vi "Restore X & Scale Indices.vi"(5 "New Plot Style in":T1, 9 "Original Plot Style in":T1) -> (8 "Updated Plot Style out":T1)   [LabVIEW 2019]
uses:
  XY Graph Plot Properties.ctl
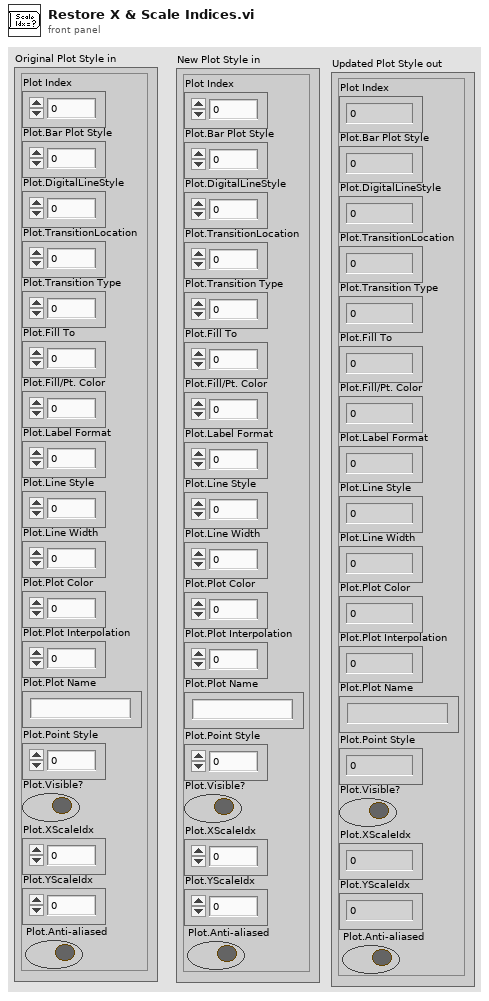
[diagram p1: front panel]
types:
  T1 = typedef "XY Graph Plot Properties.ctl" = cluster{"Plot Index":i32, "Plot.Bar Plot Style":u8, "Plot.DigitalLineStyle":u8, "Plot.TransitionLocation":u8, "Plot.Transition Type":u8, "Plot.Fill To":i16, "Plot.Fill/Pt. Color":u32, "Plot.Label Format":u8, "Plot.Line Style":u8, "Plot.Line Width":u8, "Plot.Plot Color":u32, "Plot.Plot Interpolation":u8, "Plot.Plot Name":string, "Plot.Point Style":u8, "Plot.Visible?":bool, "Plot.XScaleIdx":u32, "Plot.YScaleIdx":u32, "Plot.Anti-aliased":bool}
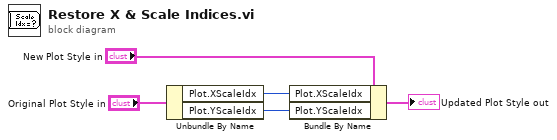
[diagram p0: block diagram]
diagram:
  n1 = Unbundle By Name("Original Plot Style in") -> ("Plot.XScaleIdx"=w2:u32, "Plot.YScaleIdx"=w1:u32)
  n2 = Bundle By Name(cluster="New Plot Style in", "Plot.XScaleIdx"=w2, "Plot.YScaleIdx"=w1) -> (→"Updated Plot Style out":T1)
